vi "Configure.vi"(8 "error in (no error)":errorcluster caption="错误输入（无错误）", 10 "Function":T1=enum."AC Current", 11 "DMM 输入":refnum<class "DMM.lvclass">) -> (0 "error out":errorcluster caption="错误输出", 3 "DMM 输出":refnum<class "DMM.lvclass">)   [LabVIEW 2020, in "DMM.lvlib" / "DMM.lvclass"]
uses:
  DMM.lvclass
  DMM.lvclass/DMM.ctl
  Function.ctl
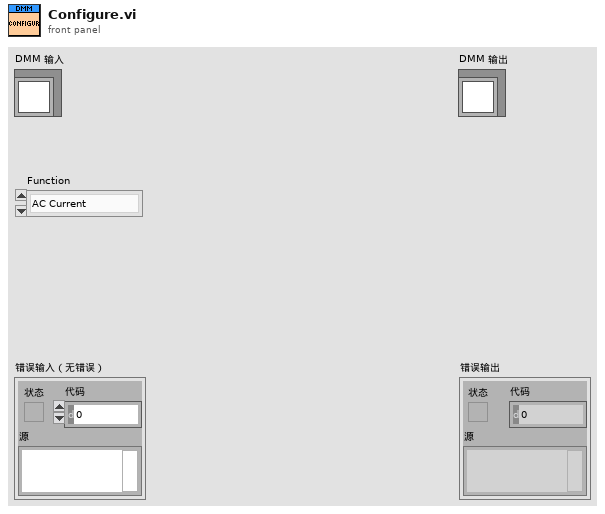
[diagram p1: front panel]
types:
  T1 = typedef "DMM.lvlib/DMM.lvclass/Function.ctl" = enum16{"DC Volts", "AC Volts", "DC Current", "AC Current", "2-Wire Resistance", "4-Wire Resistance"}
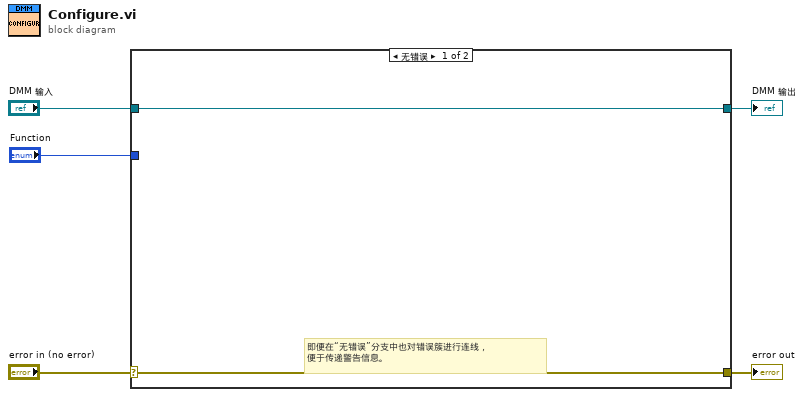
[diagram p0: block diagram]
diagram:
  n1 = case shown="无错误" "error in (no error)" {
    selector: "error in (no error)" -> [w6 w9]
    tunnel: [w6 w9] -> w4
    tunnel: [w7 w8] -> w2
    tunnel: "DMM 输入" -> [w7 w8]
    tunnel: "Function" -> [_ _]
    frame No Error {
      # "即便在“无错误”分支中也对错误簇进行连线，\n便于传递警告信息。"
    }
    frame Error {
    }
  }
  "error out" <- w4
  "DMM 输出" <- w2
